vi "Hardware Selector.vi"(8 "Error In":errorcluster, 11 "Hardware Configuration":T1) -> (0 "Error Out":errorcluster, 3 "Selected Hardware Configuration":T1)   [LabVIEW 2015]
uses:
  Hardware_Configuration.ctl
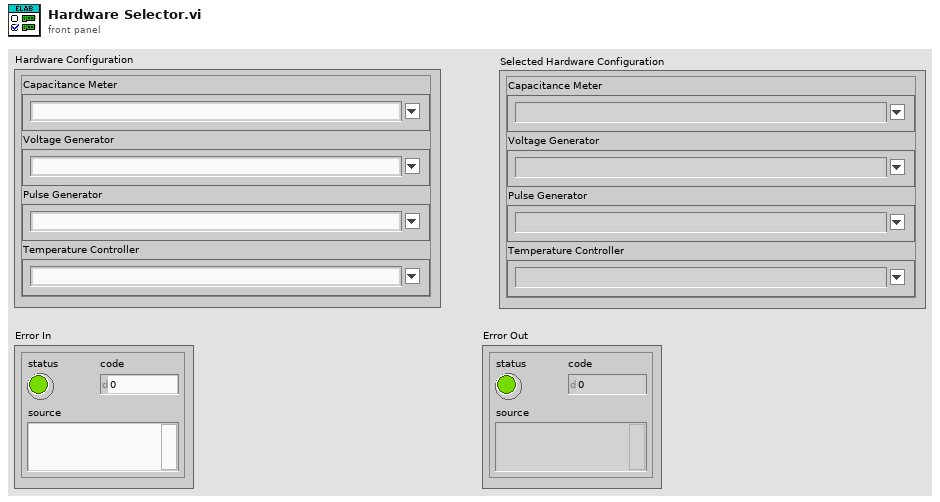
[diagram p1: front panel]
types:
  T1 = typedef "Hardware_Configuration.ctl" = cluster{"Capacitance Meter":string, "Voltage Generator":string, "Pulse Generator":string, "Temperature Controller":string}
  T2 = cluster{"Capacitance Meter":string, "Voltage Generator":string, "Pulse Generator":string, "Temperature Controller":string}
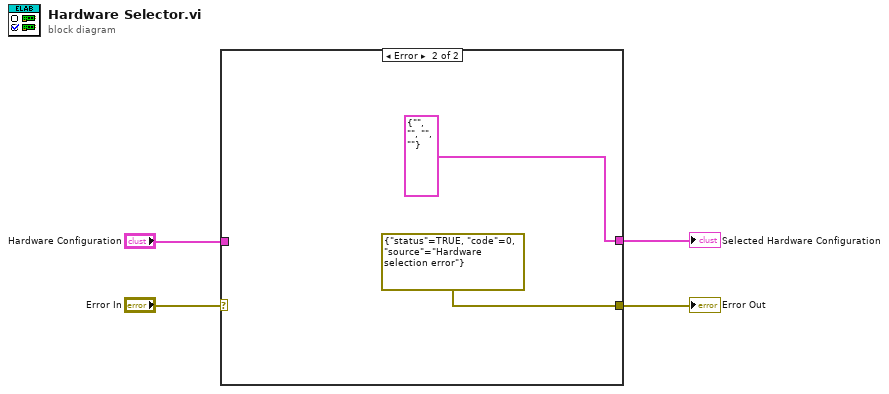
[diagram p0: block diagram]
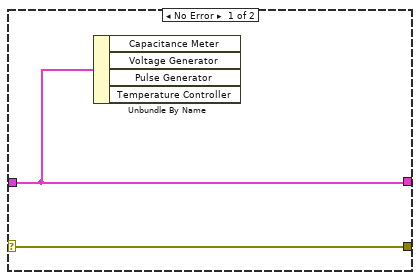
[diagram p2: hidden frame]
diagram:
  n1 = case shown="Error" "Error In" {
    selector: "Error In" -> [w6 _]
    tunnel: "Hardware Configuration" -> [w5 _]
    tunnel: [w6 errorcluster {"status"=TRUE, "code"=0, "source"="Hardware selection error"} ("error constant")] -> w2
    tunnel: [w5 T2 {"Capacitance Meter"="", "Voltage Generator"="", "Pulse Generator"="", "Temperature Controller"=""} ("Hardware Configuration")] -> w1
    frame No Error {
      n2 = Unbundle By Name(w5) -> ()  [unwired: 4 out]
    }
    frame Error {
    }
  }
  "Error Out" <- w2
  "Selected Hardware Configuration" <- w1
